vi "Simple_Initialize.vi"(7 "PwrSns Model RegEx":string, 8 "error in (no error)":errorcluster, 9 "Reset (True)":bool=TRUE, 10 "ID Query (True)":bool=TRUE, 11 "VISA resource name":refnum<visa-resource-name>) -> (0 "error out":errorcluster, 3 "VISA resource name out":refnum<visa-resource-name>)   [LabVIEW 2025, in "Interface Functions.lvlib"]
doc: "Establishes communication with the instrument and optionally performs an instrument identification query and/or an instrument reset. It also places the instrument in a default state needed for other instrument driver operations. Therefore, call this VI before calling other instrument driver VIs for this instrument. Generally, you need to call the Initialize VI only once at the beginning of an application."
uses:
  Interface Functions.lvlib
  <vilib>/regexp/Match Regular Expression.xnode
  <instrlib>/Agilent U2000 Series/Agilent U2000 Series.lvlib
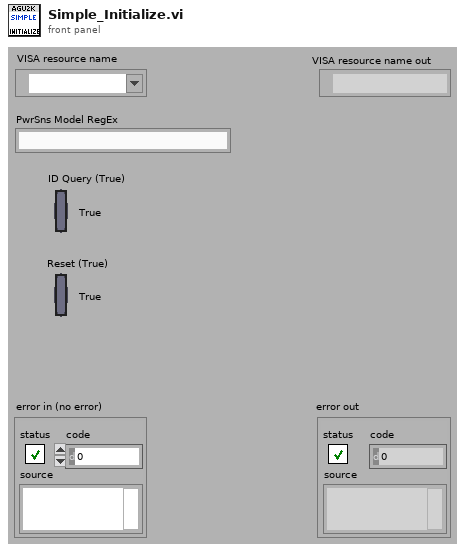
[diagram p1: front panel]
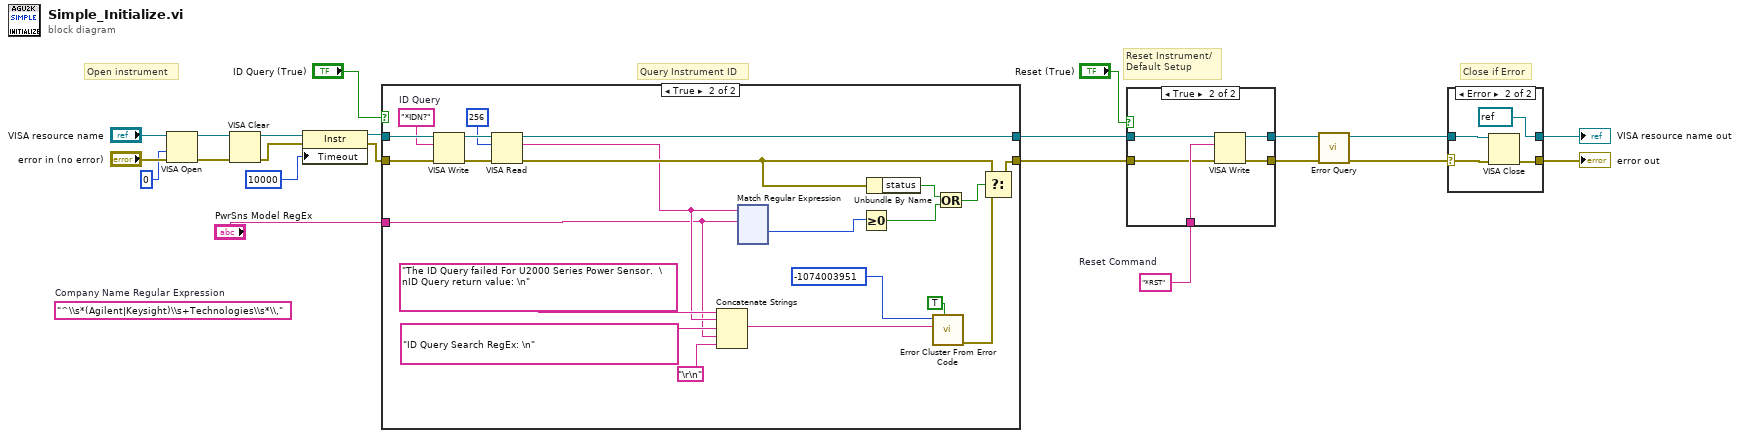
[diagram p0: block diagram]
diagram:
  (unwired) "^\\s*(Agilent|Keysight)\\s+Technologies\\s*\\,"  # Company Name Regular Expression
  w6 = "*RST"  # Reset Command
  # "Close if Error"
  # "Query Instrument ID"
  # "Reset Instrument/\nDefault Setup"
  # "Open instrument"
  n1 = VISA Open(access mode=u32 0, error in (no error)="error in (no error)", VISA resource name="VISA resource name") -> (VISA resource name=w17:refnum<visa-resource-name>, error out=w16:errorcluster)  [unwired: 2 out]
  n2 = VISA Clear(VISA resource name=w17, error in (no error)=w16) -> (VISA resource name out=w13:refnum<visa-resource-name>, error out=w12:errorcluster)
  n3 = property class="Instr"(reference=w13, error in=w12, "Timeout"=u32 10000 ("General Settings:Timeout Value")) -> (reference out=w10:refnum<visa-resource-name>, error out=w9:errorcluster)
  n4 = case shown="True" "ID Query (True)" {
    tunnel: [w23 w46] -> w7
    tunnel: [w24 w43] -> w8
    tunnel: w10 -> [w24 w44]
    tunnel: w9 -> [w23 w45]
    tunnel: "PwrSns Model RegEx" -> [_ w27]
    frame False {
    }
    frame True {
      w39 = "*IDN?"  # ID Query
      n5 = VISA Write(VISA resource name=w44, write buffer=w39, error in (no error)=w45) -> (VISA resource name out=w42:refnum<visa-resource-name>, error out=w41:errorcluster)  [unwired: 1 out]
      n6 = VISA Read(VISA resource name=w42, byte count=u32 256, error in (no error)=w41) -> (VISA resource name out=w43:refnum<visa-resource-name>, read buffer=w29:string, error out=w35:errorcluster)  [unwired: 1 out]
      n7 = Concatenate Strings("The ID Query failed For U2000 Series Power Sensor.  \nID Query return value: \n" ("Source (VI Name)"), w29, "ID Query Search RegEx: \n" ("Source (VI Name)"), w27, "\r\n") -> (w25:string)
      n8 = xnode "Match Regular Expression"("input string"=w29, "regular expression"=w27) -> ("offset past match"=w31:i32)  [unwired: 4 in, 4 out]
      n9 = Greater Or Equal To 0?(x=w31) -> (x >= 0?=w33:bool)
      n10 = Unbundle By Name(w35) -> ("status"=w34:bool)
      n11 = call <vilib>:"Error Cluster From Error Code.vi"("show call chain? (False)"=TRUE, "error message (\"\")"=w25, "error code (0)"=-1074003951 ("Code")) -> ("error out"=w38:errorcluster)  [unwired: 1 in, 5 out]
      n12 = Or(x=w34, y=w33) -> (x .or. y?=w32:bool)
      n13 = Select(t=w35, s=w32, f=w38) -> (s? t:f=w46:errorcluster)
    }
  }
  n14 = case shown="True" "Reset (True)" {
    tunnel: w7 -> [w164 w167]
    tunnel: [w164 w169] -> w4
    tunnel: w8 -> [w165 w166]
    tunnel: [w165 w170] -> w5
    tunnel: w6 -> [_ w168]
    frame False {
    }
    frame True {
      n15 = VISA Write(VISA resource name=w166, write buffer=w168, error in (no error)=w167) -> (VISA resource name out=w170:refnum<visa-resource-name>, error out=w169:errorcluster)  [unwired: 1 out]
    }
  }
  n16 = call <instrlib>:"Error Query.vi"("error in (no error)"=w4, "VISA resource name"=w5) -> ("error out"=w2:errorcluster, "VISA resource name out"=w3:refnum<visa-resource-name>)  [unwired: 8 out]
  n17 = case shown="Error" w2 {
    selector: w2 -> [w171 w174]
    tunnel: w3 -> [w172 w175]
    tunnel: [w172 refnum<visa-resource-name> refnum ("VISA resource name out")] -> w15
    tunnel: [w171 w173] -> w14
    frame No Error {
    }
    frame Error {
      n18 = VISA Close(VISA resource name=w175, error in (no error)=w174) -> (error out=w173:errorcluster)
    }
  }
  "VISA resource name out" <- w15
  "error out" <- w14
